vi "Set Window.vi"(8 "error in (no error)":errorcluster, 9 "Cluster":T1, 11 "Refnum in":refnum<k20>) -> (0 "error out":errorcluster, 3 "Refnum out":refnum<k20>)   [LabVIEW 2013]
uses:
  Cluser.ctl
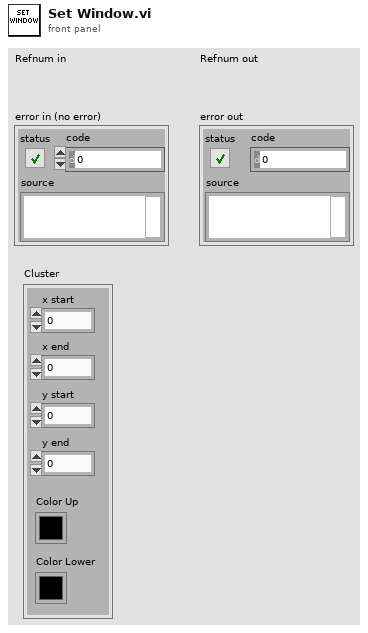
[diagram p1: front panel]
types:
  T1 = typedef "Cluser.ctl" = cluster{"x start":u16, "x end":u16, "y start":u16, "y end":u16, "Color Up":u32, "Color Lower":u32}
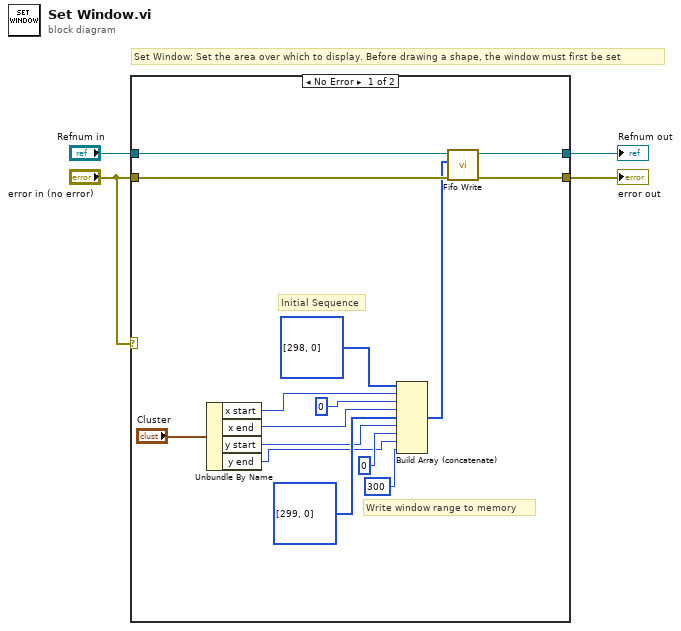
[diagram p0: block diagram]
diagram:
  # "Set Window: Set the area over which to display. Before drawing a shape, the window must first be set"
  n1 = case shown="No Error" "error in (no error)" {
    tunnel: [w19 w20] -> w4
    tunnel: [w18 w21] -> w3
    tunnel: "error in (no error)" -> [w17 w20]
    tunnel: "Refnum in" -> [w16 w21]
    frame No Error {
      # "Write window range to memory"
      # "Initial Sequence"
      n2 = Unbundle By Name("Cluster") -> ("x start"=w13:u16, "x end"=w11:u16, "y start"=w9:u16, "y end"=w7:u16)
      n3 = Build Array (concatenate)(u16[] [298, 0], w13, u16 0 ("element"), w11, u16[] [299, 0], w9, u16 0 ("element"), w7, u16 300 ("element")) -> (w5:u16[])
      n4 = call "Fifo Write.vi"("error in (no error)"=w17, "Data"=w5, "Refnum in"=w16) -> ("error out"=w19:errorcluster, "Refnum out"=w18:refnum<k20>)  [unwired: 7 in]
    }
    frame Error {
    }
  }
  "error out" <- w4
  "Refnum out" <- w3
